vi "BackupFile.vi"(11 "path in":path) -> (0 "error out":errorcluster, 3 "path out":path)   [LabVIEW 2025]
uses:
  <vilib>/Utility/error.llb/DialogType.ctl
panel:
  out "SelectErrorTst":string
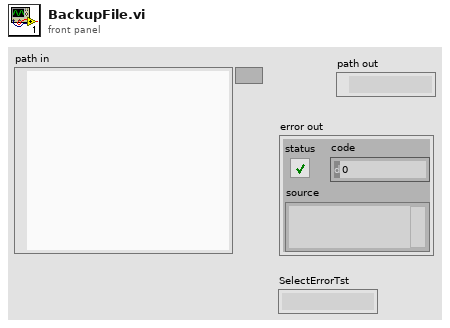
[diagram p1: front panel]
types:
  T1 = typedef "DialogType.ctl" = u16
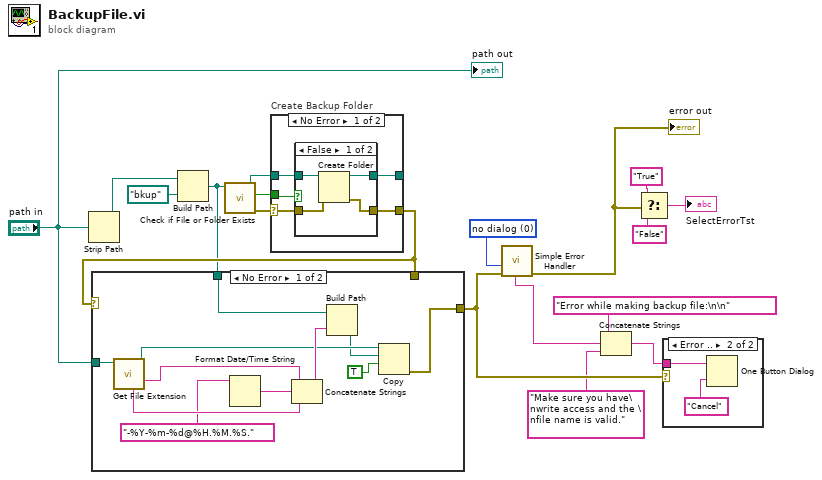
[diagram p0: block diagram]
diagram:
  w6 = T1 0 items=["no dialog", "OK message", "continue or stop message", "OK message + warnings", "continue/stop + warnings"] ("type of dialog (OK msg:1)")
  n1 = Strip Path(path="path in") -> (stripped path=w18:path)  [unwired: 1 out]
  n2 = Build Path(base path=w18, name or relative path=path "bkup") -> (appended path=w8:path)
  n3 = call <vilib>:"Check if File or Folder Exists.vi"("path"=w8) -> ("error out"=w16:errorcluster, "file or folder exists?"=w15:bool, "dup path"=w14:path)  [unwired: 8 in]
  n4 = case "Create Backup Folder" shown="No Error" w16 {
    selector: w16 -> [w21 w31]
    tunnel: w15 -> [w23 _]
    tunnel: w14 -> [w22 w30]
    tunnel: [w19 w31] -> w10
    tunnel: [w20 w30] -> _
    frame No Error {
      n5 = case shown="False" w23 {
        tunnel: w22 -> [w27 w28]
        tunnel: [w26 w28] -> w20
        tunnel: [w25 w29] -> w19
        tunnel: w21 -> [w24 w29]
        frame False {
          n6 = Create Folder(path (use dialog)=w27, error in=w24) -> (created path=w26:path, error out=w25:errorcluster)  [unwired: 1 in, 1 out]
        }
        frame True {
        }
      }
    }
    frame Error {
    }
  }
  n7 = case shown="No Error" w10 {
    tunnel: [w37 w43] -> w5
    tunnel: w10 -> [_ w43]
    tunnel: "path in" -> [w42 _]
    tunnel: w8 -> [w39 _]
    frame No Error {
      n8 = call <vilib>:"Get File Extension.vi"("file"=w42) -> ("filename without extension"=w41:string, "dup file"=w36:path, "unmodified file extension"=w40:string)  [unwired: 6 in, 2 out]
      n9 = Format Date/Time String(time format string (%c)="-%Y-%m-%d@%H.%M.%S.") -> (date/time string=w33:string)  [unwired: 2 in]
      n10 = Concatenate Strings(w41, w33, w40) -> (w38:string)
      n11 = Build Path(base path=w39, name or relative path=w38) -> (appended path=w35:path)
      n12 = Copy(9:TRUE ("overwrite (F)"), 10:w35, 11:w36) -> (0:w37:errorcluster)  [unwired: 2 in, 2 out]
    }
    frame Error {
    }
  }
  n13 = call <vilib>:"Simple Error Handler.vi"("type of dialog (OK msg:1)"=w6, "error in (no error)"=w5) -> ("error out"=w7:errorcluster, "message"=w2:string)  [unwired: 3 in, 3 out]
  "error out" <- w7
  n14 = Concatenate Strings("Error while making backup file:\n\n", w2, "Make sure you have\nwrite access and the \nfile name is valid." ("string")) -> (w3:string)
  n15 = Select(t="True", s=w7, f="False") -> (s? t:f=→"SelectErrorTst":string)
  n16 = case shown="Error .." w5 {
    tunnel: w3 -> [_ w45]
    frame No Error {
    }
    frame Error {
      n17 = One Button Dialog(message=w45, button name ("OK")="Cancel") -> ()  [unwired: 1 out]
    }
  }
  "path out" <- "path in"
